vi "ReadSweep.vi"(8 "error in (no error)":errorcluster, 11 "9770 API in":refnum<class "9770 API.lvclass">) -> (0 "error out":errorcluster, 1 "sweep valid":bool, 2 "sweep":cluster{"frequency":dbl, "amplitude":dbl}[](array[cluster]), 3 "9770 API out":refnum<class "9770 API.lvclass">, 4 "sweep time (seconds)":dbl, 5 "ChannelName":string, 6 "current sweep frequency":dbl, 7 "Units":string)   [LabVIEW 2017, in "9770 API.lvclass"]
uses:
  <vilib>/addons/InsightCM/Devices/Shared/Emsa/Emsa9770API/9770 API.lvclass
  <vilib>/addons/InsightCM/Devices/Shared/Emsa/Emsa9770API/9770 API.lvclass/9770 API.ctl
  <vilib>/LabVIEW Targets/FPGA/cRIO/shared/nicrio_ModuleControls/nicrio_cRIO-9770_DataRatesRing.ctl
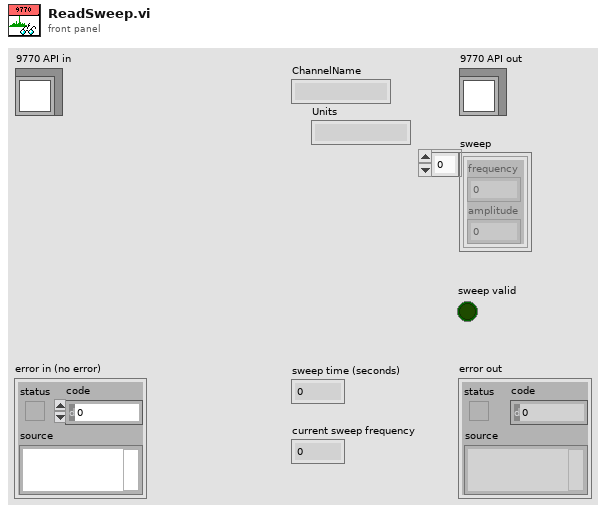
[diagram p1: front panel]
types:
  T1 = cluster{"Sweep":cluster{"Center Freq":dbl, "Bandwidth":dbl}[], "SampleRate":dbl, "FullScaleVoltage":dbl, "DetectionTime":dbl, "DetectionMode":enum16{"Peak", "Quasi Peak", "Average"}}
  T2 = typedef "nicrio_cRIO-9770_DataRatesRing.ctl" = u8
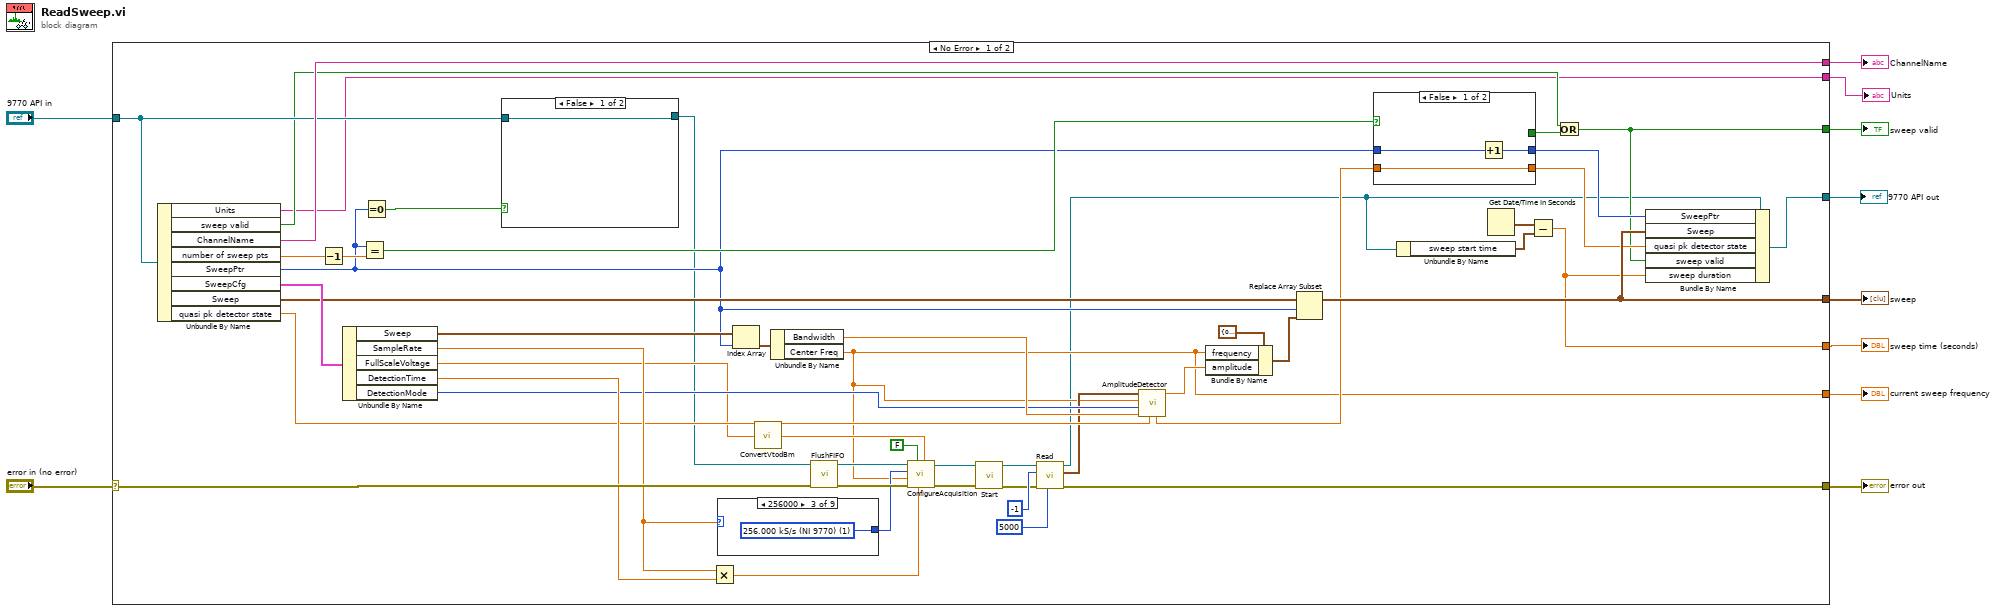
[diagram p0: block diagram]
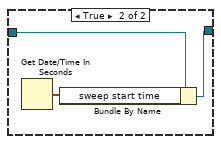
[diagram p2: hidden frame]
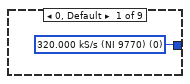
[diagram p3: hidden frame]
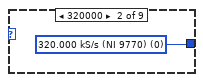
[diagram p4: hidden frame]
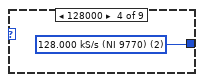
[diagram p5: hidden frame]
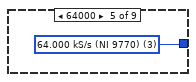
[diagram p6: hidden frame]
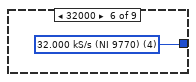
[diagram p7: hidden frame]
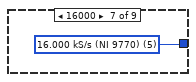
[diagram p8: hidden frame]
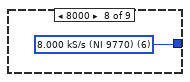
[diagram p9: hidden frame]
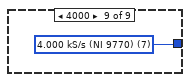
[diagram p10: hidden frame]
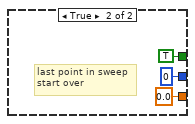
[diagram p11: hidden frame]
diagram:
  n1 = case shown="No Error" "error in (no error)" {
    selector: "error in (no error)" -> [w60 w81]
    tunnel: [w35 w81] -> w9
    tunnel: [w31 w80] -> w7
    tunnel: "9770 API in" -> [w24 w80]
    tunnel: [w21 _] -> w6
    tunnel: [w36 _] -> w5
    tunnel: [w27 _] -> w4
    tunnel: [w15 _] -> w3
    tunnel: [w18 _] -> w2
    tunnel: [w13 _] -> w1
    frame No Error {
      n2 = Unbundle By Name(w24) -> ("Units"=w13:string, "sweep valid"=w20:bool, "ChannelName"=w27:string, "number of sweep pts"=w42:dbl, "SweepPtr"=w26:i32, "SweepCfg"=w57:T1, "Sweep"=w40:cluster{"frequency":dbl, "amplitude":dbl}[], "quasi pk detector state"=w34:dbl)
      n3 = Decrement(x=w42) -> (x-1=w41:dbl)
      n4 = Unbundle By Name(w57) -> ("Sweep"=w55:cluster{"Center Freq":dbl, "Bandwidth":dbl}[], "SampleRate"=w50:dbl, "FullScaleVoltage"=w29:dbl, "DetectionTime"=w53:dbl, "DetectionMode"=w43:enum16{"Peak", "Quasi Peak", "Average"})
      n5 = Equal?(x=w26, y=w41) -> (x = y?=w37:bool)
      n6 = Equal To 0?(x=w26) -> (x = 0?=w25:bool)
      n7 = case shown="False" w25 {
        tunnel: w24 -> [w61 w64]
        tunnel: [w61 w63] -> w23
        frame False {
        }
        frame True {
          n8 = Get Date/Time In Seconds() -> (seconds since 1Jan1904=w62:timestamp)
          n9 = Bundle By Name(cluster=w64, "sweep start time"=w62) -> (w63:refnum<class "9770 API.lvclass">)
        }
      }
      n10 = Multiply(x=w50, y=w53) -> (x*y=w52:dbl)
      n11 = case shown="256000" w50 {
        tunnel: [w65 w66 w67 w68 w69 w70 w71 w72 w73] -> w51
        frame 0, Default {
          w65 = T2 0 items=["320.000 kS/s (NI 9770)", "256.000 kS/s (NI 9770)", "128.000 kS/s (NI 9770)", "64.000 kS/s (NI 9770)", "32.000 kS/s (NI 9770)", "16.000 kS/s (NI 9770)", "8.000 kS/s (NI 9770)", "4.000 kS/s (NI 9770)"] ("Data Rate")
        }
        frame 320000 {
          w66 = T2 0 items=["320.000 kS/s (NI 9770)", "256.000 kS/s (NI 9770)", "128.000 kS/s (NI 9770)", "64.000 kS/s (NI 9770)", "32.000 kS/s (NI 9770)", "16.000 kS/s (NI 9770)", "8.000 kS/s (NI 9770)", "4.000 kS/s (NI 9770)"] ("Data Rate")
        }
        frame 256000 {
          w67 = T2 1 items=["320.000 kS/s (NI 9770)", "256.000 kS/s (NI 9770)", "128.000 kS/s (NI 9770)", "64.000 kS/s (NI 9770)", "32.000 kS/s (NI 9770)", "16.000 kS/s (NI 9770)", "8.000 kS/s (NI 9770)", "4.000 kS/s (NI 9770)"] ("Data Rate")
        }
        frame 128000 {
          w68 = T2 2 items=["320.000 kS/s (NI 9770)", "256.000 kS/s (NI 9770)", "128.000 kS/s (NI 9770)", "64.000 kS/s (NI 9770)", "32.000 kS/s (NI 9770)", "16.000 kS/s (NI 9770)", "8.000 kS/s (NI 9770)", "4.000 kS/s (NI 9770)"] ("Data Rate")
        }
        frame 64000 {
          w69 = T2 3 items=["320.000 kS/s (NI 9770)", "256.000 kS/s (NI 9770)", "128.000 kS/s (NI 9770)", "64.000 kS/s (NI 9770)", "32.000 kS/s (NI 9770)", "16.000 kS/s (NI 9770)", "8.000 kS/s (NI 9770)", "4.000 kS/s (NI 9770)"] ("Data Rate")
        }
        frame 32000 {
          w70 = T2 4 items=["320.000 kS/s (NI 9770)", "256.000 kS/s (NI 9770)", "128.000 kS/s (NI 9770)", "64.000 kS/s (NI 9770)", "32.000 kS/s (NI 9770)", "16.000 kS/s (NI 9770)", "8.000 kS/s (NI 9770)", "4.000 kS/s (NI 9770)"] ("Data Rate")
        }
        frame 16000 {
          w71 = T2 5 items=["320.000 kS/s (NI 9770)", "256.000 kS/s (NI 9770)", "128.000 kS/s (NI 9770)", "64.000 kS/s (NI 9770)", "32.000 kS/s (NI 9770)", "16.000 kS/s (NI 9770)", "8.000 kS/s (NI 9770)", "4.000 kS/s (NI 9770)"] ("Data Rate")
        }
        frame 8000 {
          w72 = T2 6 items=["320.000 kS/s (NI 9770)", "256.000 kS/s (NI 9770)", "128.000 kS/s (NI 9770)", "64.000 kS/s (NI 9770)", "32.000 kS/s (NI 9770)", "16.000 kS/s (NI 9770)", "8.000 kS/s (NI 9770)", "4.000 kS/s (NI 9770)"] ("Data Rate")
        }
        frame 4000 {
          w73 = T2 7 items=["320.000 kS/s (NI 9770)", "256.000 kS/s (NI 9770)", "128.000 kS/s (NI 9770)", "64.000 kS/s (NI 9770)", "32.000 kS/s (NI 9770)", "16.000 kS/s (NI 9770)", "8.000 kS/s (NI 9770)", "4.000 kS/s (NI 9770)"] ("Data Rate")
        }
      }
      n12 = Index Array(array=w55, index=w26) -> (element=w54:cluster{"Center Freq":dbl, "Bandwidth":dbl})
      n13 = call <vilib>:"ConvertVtodBm.vi"("voltage"=w29) -> ("dBm"=w28:dbl)  [unwired: 4 in]
      n14 = Unbundle By Name(w54) -> ("Bandwidth"=w44:dbl, "Center Freq"=w18:dbl)
      n15 = call <vilib>:"FlushFIFO.vi"("error in (no error)"=w60, "9770 API in"=w23) -> ("error out"=w59:errorcluster, "9770 API out"=w58:refnum<class "9770 API.lvclass">)  [unwired: 8 in]
      n16 = call <vilib>:"ConfigureAcquisition.vi"("Reference Level (dBm)"=w28, "Number of Samples"=w52, "Continuous"=FALSE, "error in (no error)"=w59, "Center Frequency (Hz)"=w18, "Data Rate"=w51, "9770 API in"=w58) -> ("error out"=w49:errorcluster, "9770 API out"=w48:refnum<class "9770 API.lvclass">)  [unwired: 3 in]
      n17 = call-dynamic "Start.vi"("error in (no error)"=w49, "RIO_API in"=w48) -> ("error out"=w11:errorcluster, "RIO_API out"=w47:refnum<class "9770 API.lvclass">)  [unwired: 8 in]
      n18 = call <vilib>:"Read.vi"("timeout (ms)"=5000, "error in (no error)"=w11, "number of samples"=-1, "9770 API in"=w47) -> ("error out"=w35:errorcluster, "Waveform"=w19:waveform(cdb), "9770 API out"=w14:refnum<class "9770 API.lvclass">)  [unwired: 2 in, 3 out]
      n19 = call <vilib>:"AmplitudeDetector.vi"("quasi peak detector in"=w34, "resolution bandwidth"=w44, "DetectionMode"=w43, "frequency"=w18, "waveform"=w19) -> ("Value"=w30:dbl, "quasi peak detector out"=w33:dbl)  [unwired: 4 in, 1 out]
      n20 = Bundle By Name(cluster=cluster{"frequency":dbl, "amplitude":dbl} {"frequency"=0.0, "amplitude"=0.0} ("new element/subarray"), "frequency"=w18, "amplitude"=w30) -> (w38:cluster{"frequency":dbl, "amplitude":dbl})
      n21 = Replace Array Subset(array=w40, new element=w38, index=w26) -> (w36:cluster{"frequency":dbl, "amplitude":dbl}[])
      n22 = case shown="False" w37 {
        tunnel: [w76 0] -> w45
        tunnel: w26 -> [w75 _]
        tunnel: w33 -> [w74 _]
        tunnel: [w74 0.0 ("quasi peak detector out")] -> w32
        tunnel: [_ TRUE] -> w22
        frame False {
          n23 = Increment(x=w75) -> (x+1=w76:i32)
        }
        frame True {
          # "last point in sweep\nstart over"
        }
      }
      n24 = Unbundle By Name(w14) -> ("sweep start time"=w17:timestamp)
      n25 = Get Date/Time In Seconds() -> (seconds since 1Jan1904=w16:timestamp)
      n26 = Subtract(x=w16, y=w17) -> (x-y=w15:dbl)
      n27 = Or(x=w20, y=w22) -> (x .or. y?=w21:bool)
      n28 = Bundle By Name(cluster=w14, "SweepPtr"=w45, "Sweep"=w36, "quasi pk detector state"=w32, "sweep valid"=w21, "sweep duration"=w15) -> (w31:refnum<class "9770 API.lvclass">)
    }
    frame Error {
    }
  }
  "error out" <- w9
  "9770 API out" <- w7
  "sweep valid" <- w6
  "sweep" <- w5
  "ChannelName" <- w4
  "sweep time (seconds)" <- w3
  "current sweep frequency" <- w2
  "Units" <- w1
